vi "DisplayEndo.vi"(4 "Init?":bool, 5 "Hand Field Force":dbl[](array[numeric]), 6 "ClosePt":dbl[](array[numeric]), 7 "Tip Field Force":dbl[](array[numeric]), 8 "AnkleTraj":dbl[][](array[numeric]), 9 "Path Via Points":dbl[][](array[numeric])=[[0.0, 0.0, 0.0], [0.0, 0.0, 0.0], [0.0, 0.0, 0.0]], 10 "Joint Coord in GCS":dbl[][](array[numeric]), 11 "3D graph in":refnum<k7>) -> (3 "3D graph out":refnum<k7>)   [LabVIEW 2014]
uses:
  <vilib>/Platform/NI_3dgraph.lvlib
  <vilib>/ptbypt/NI_PtbyPt.lvlib
panel:
  in  "sample length":i32=100
  out "LastPlotNum":i32=1
  out "error out":errorcluster
  in  "error in (no error)":errorcluster
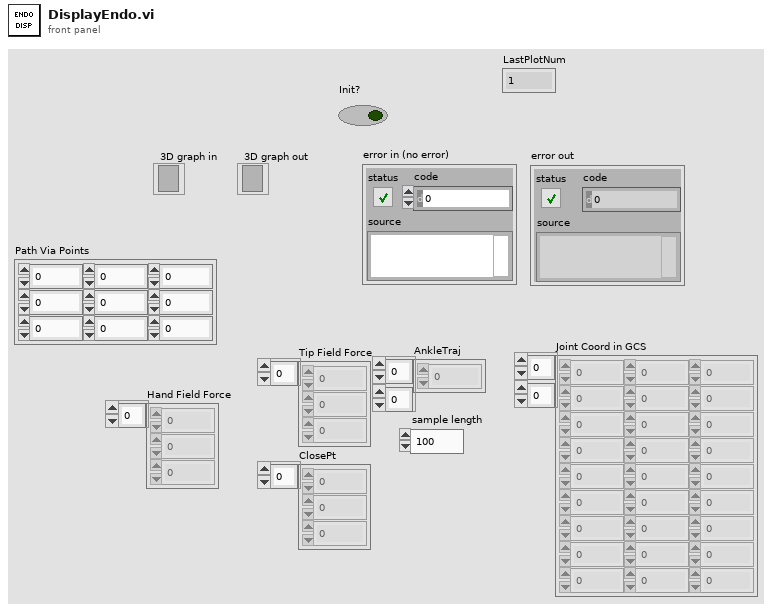
[diagram p1: front panel]
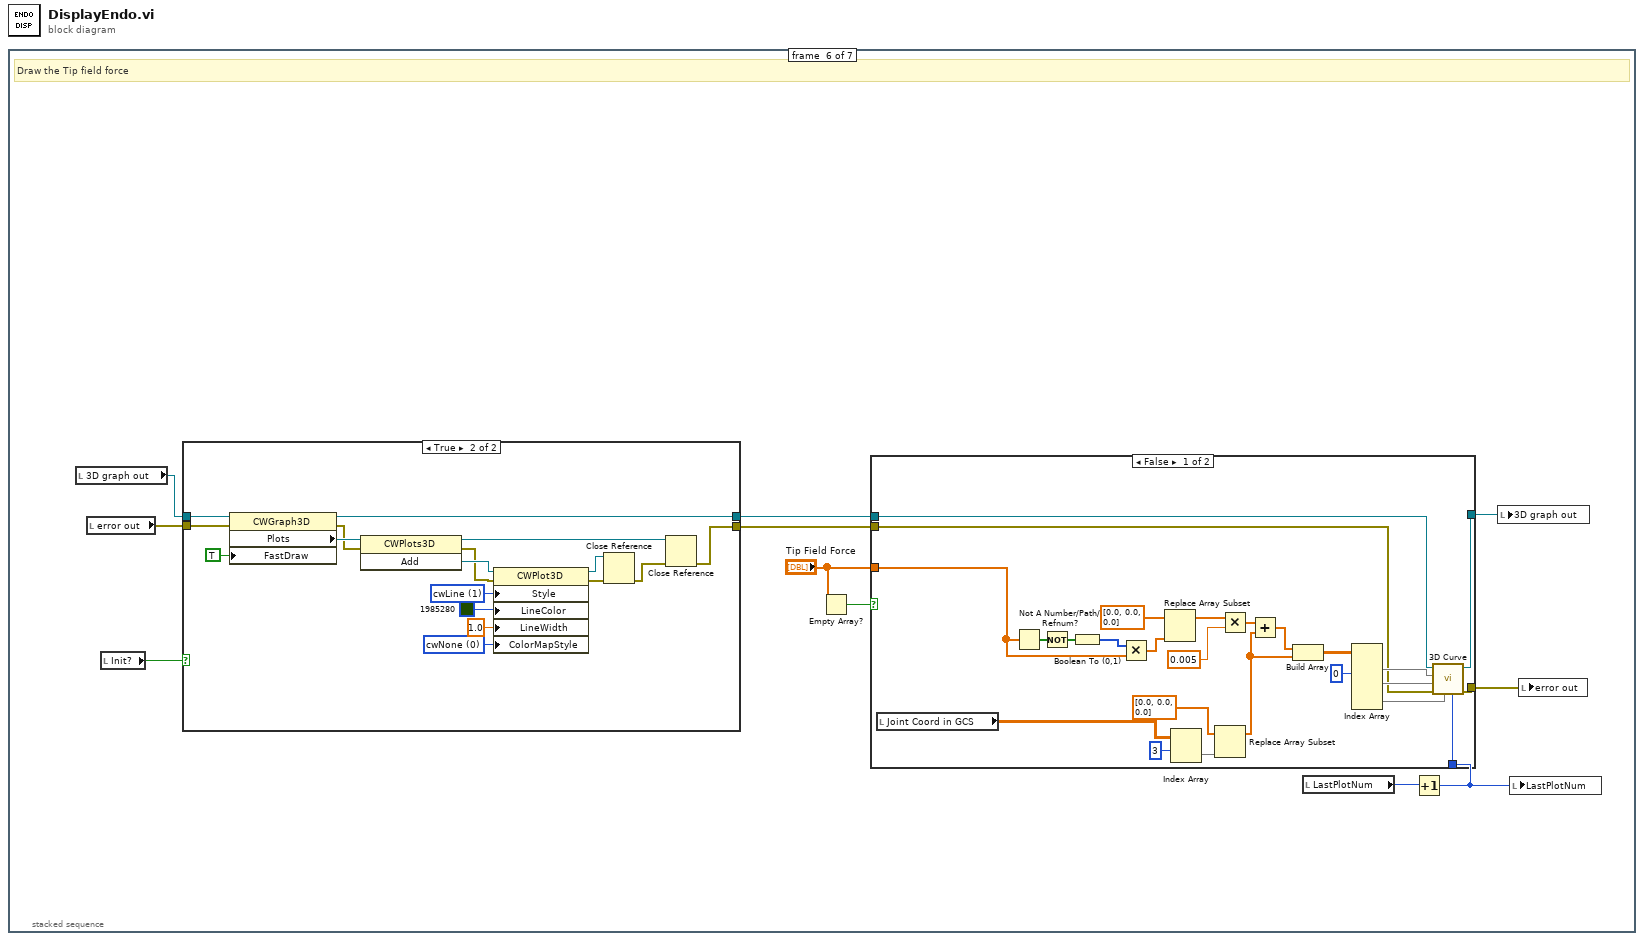
[diagram p0: block diagram]
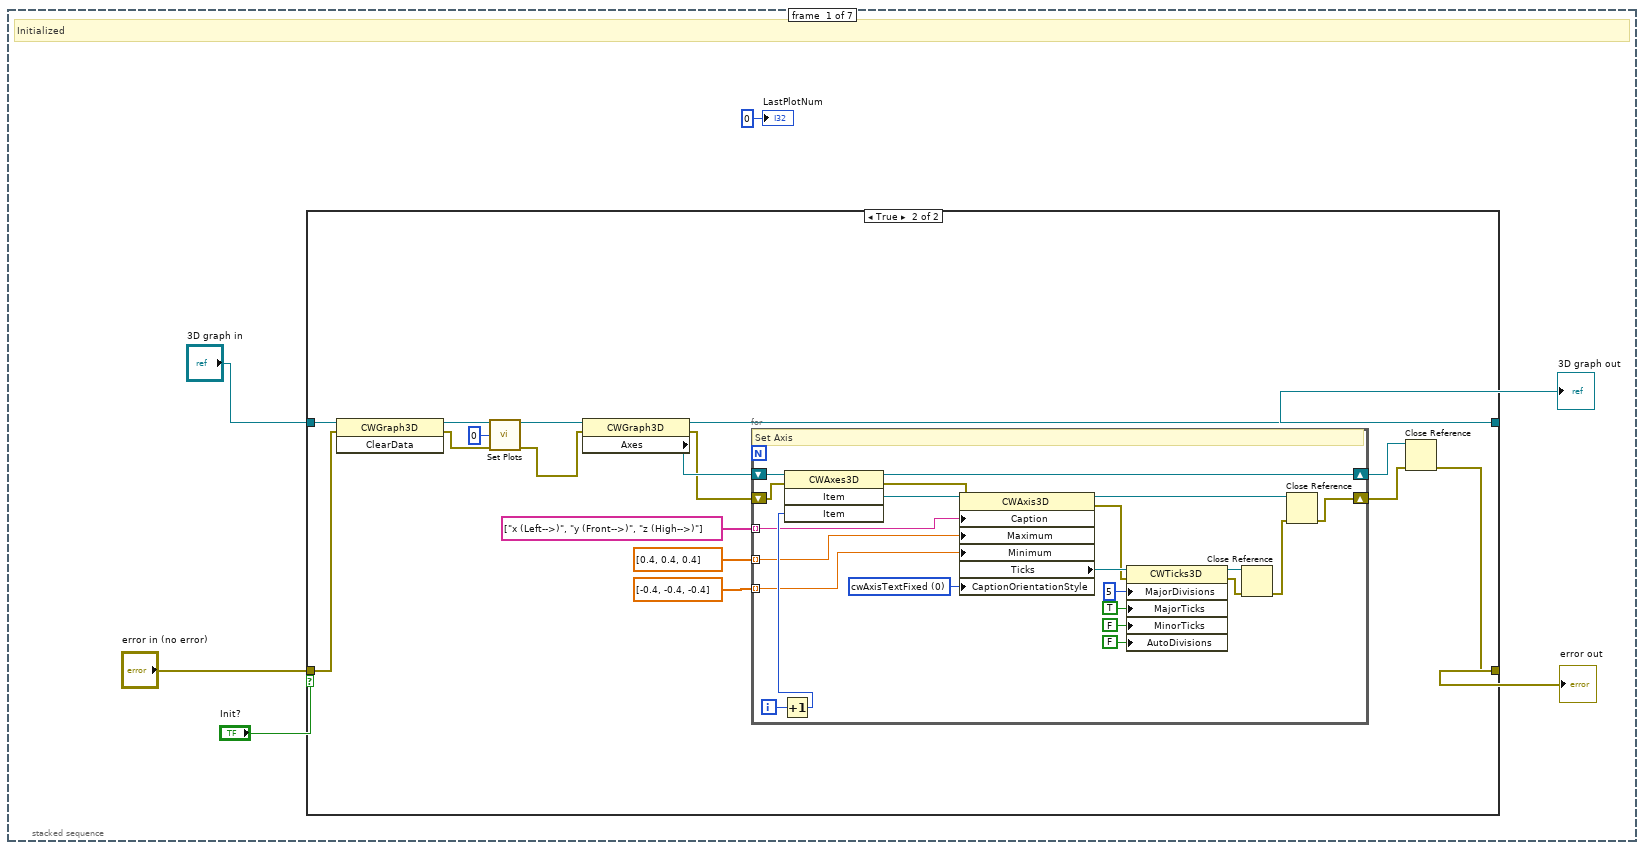
[diagram p2: hidden frame]
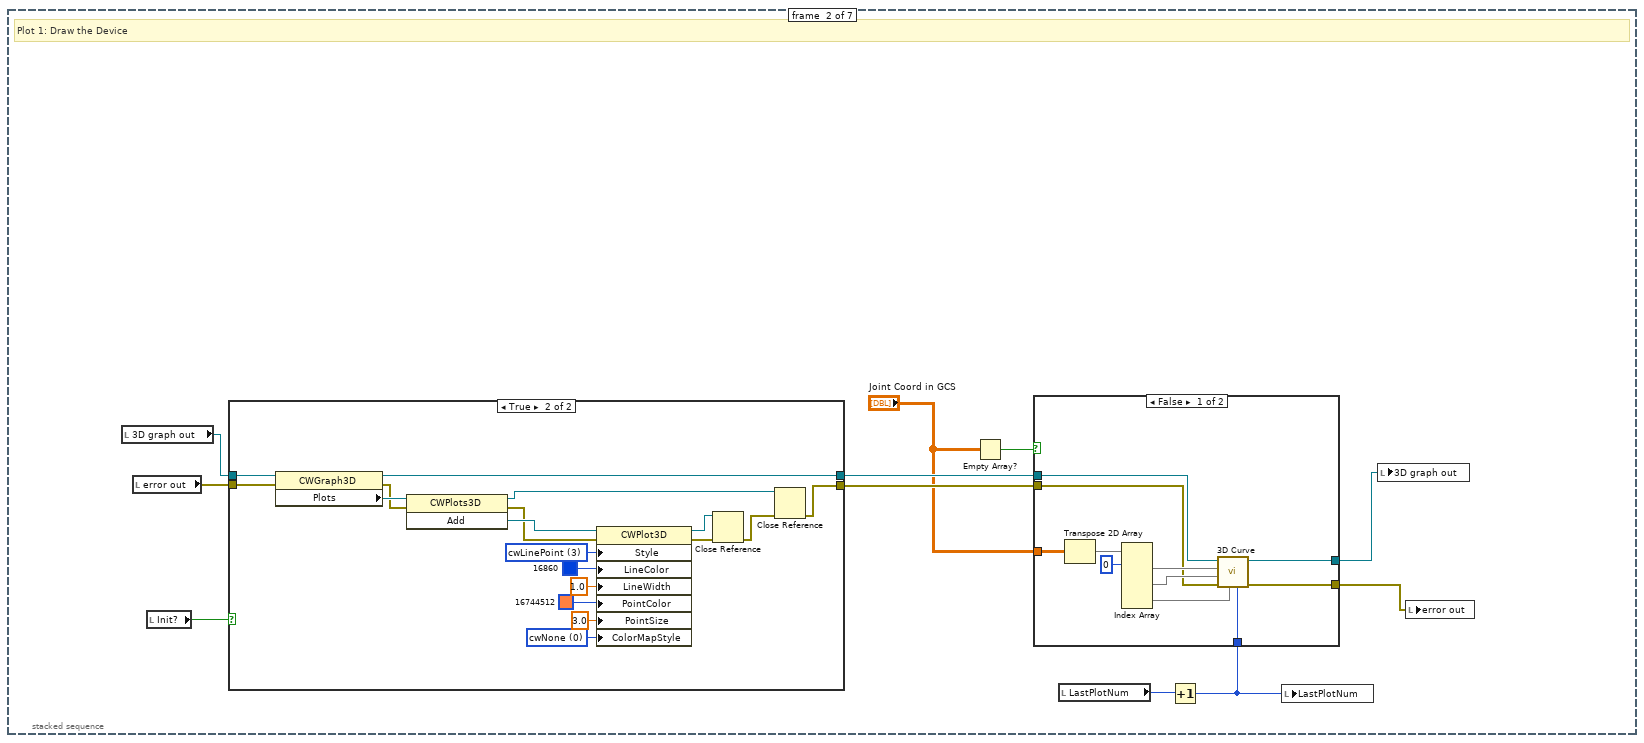
[diagram p4: hidden frame]
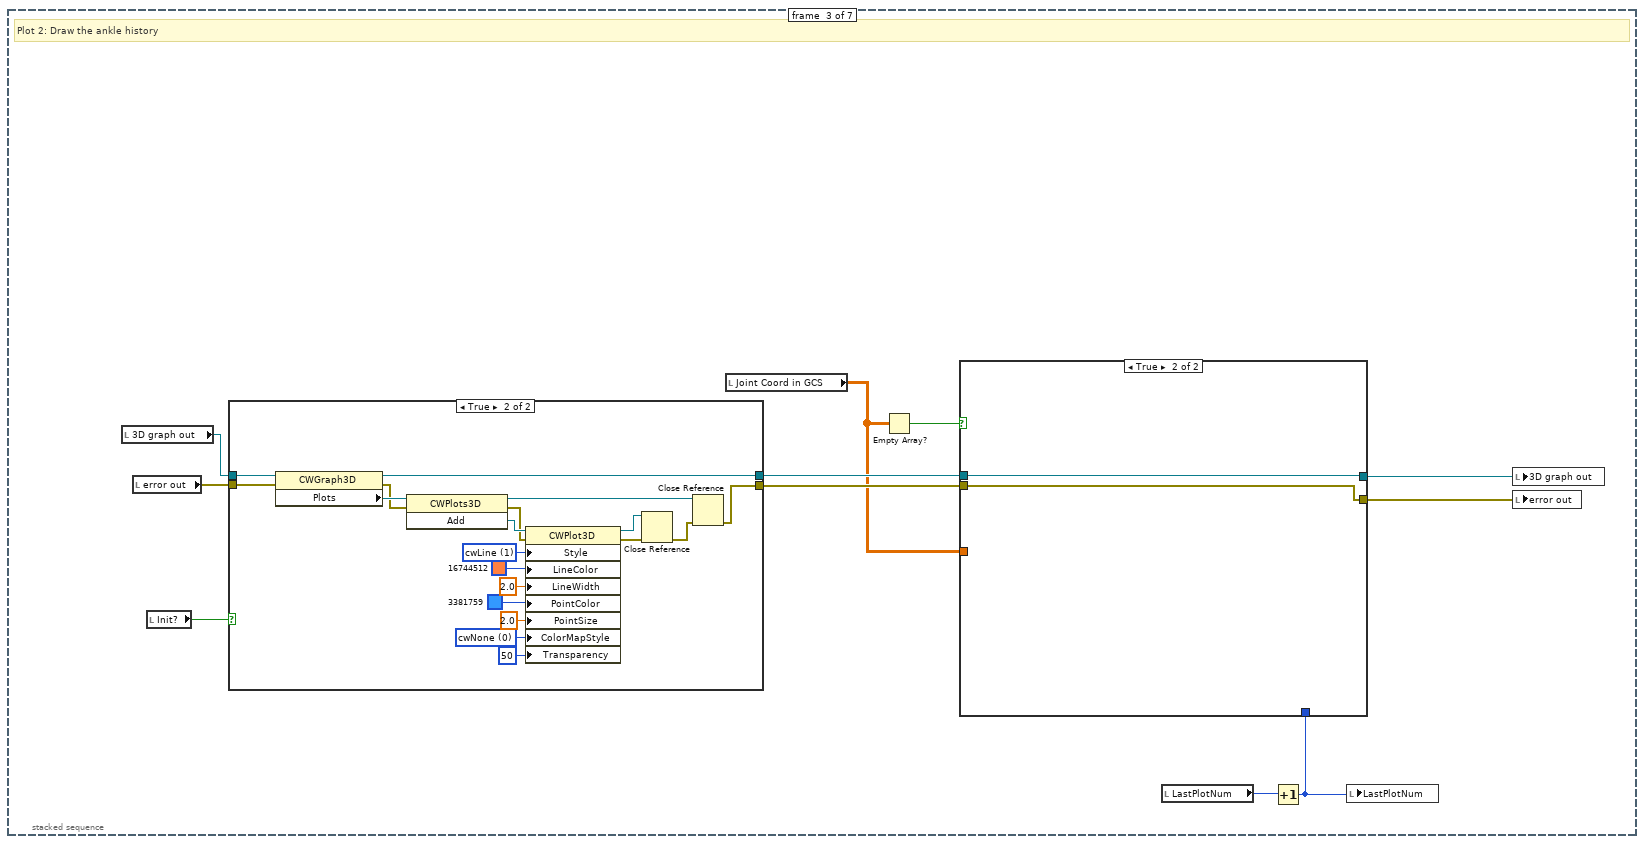
[diagram p7: hidden frame]
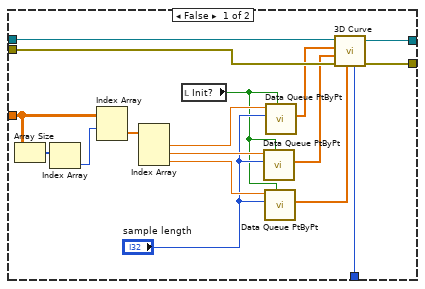
[diagram p8: hidden frame]
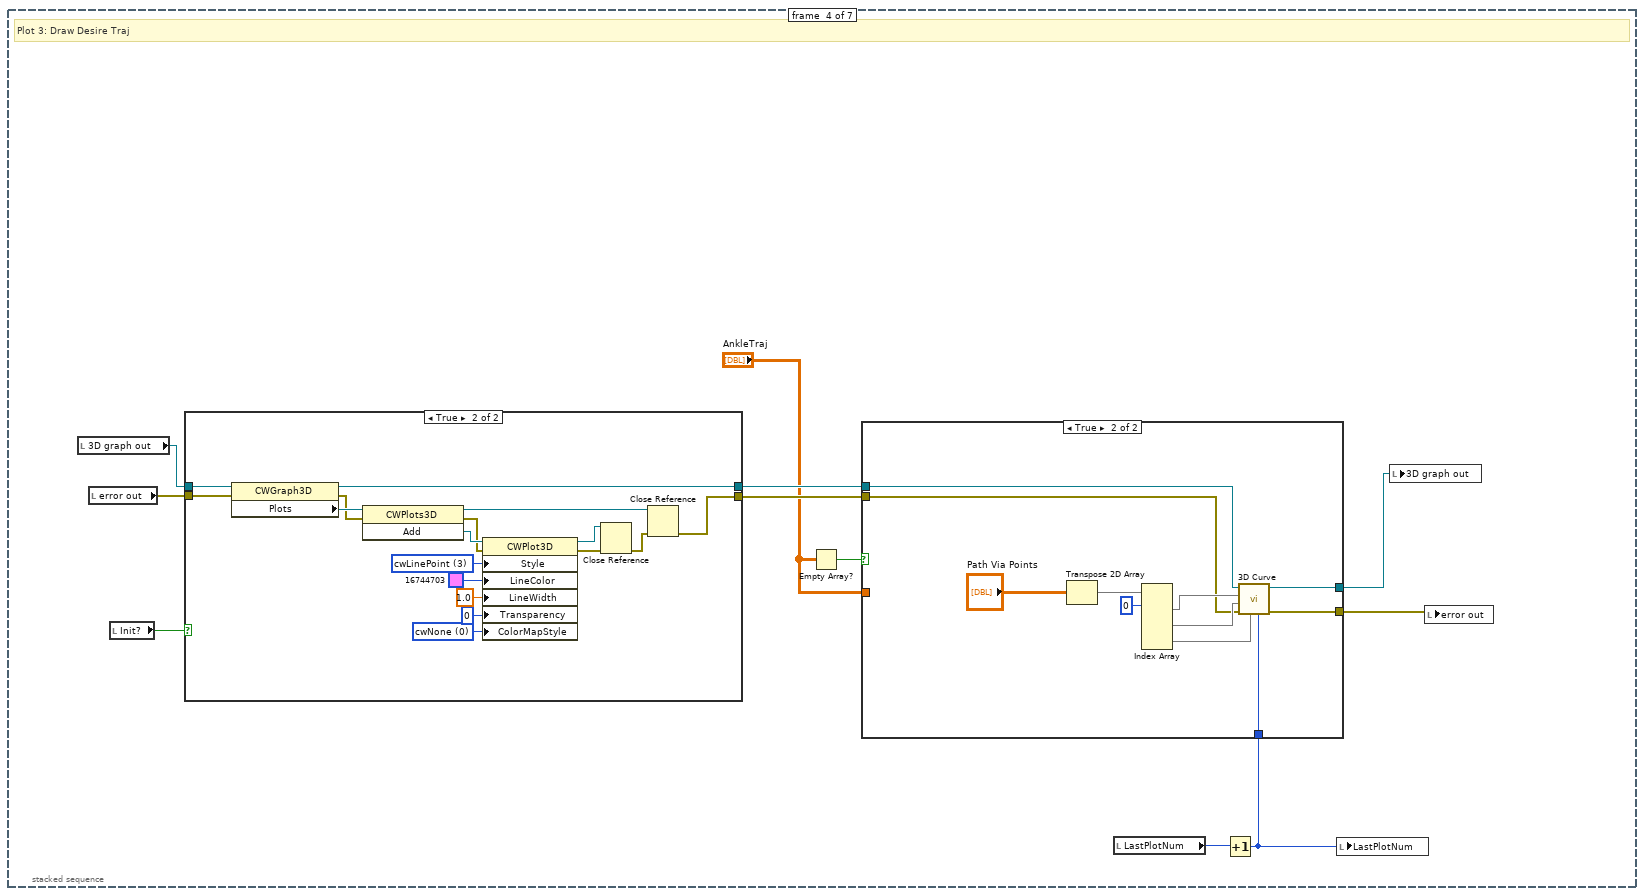
[diagram p10: hidden frame]
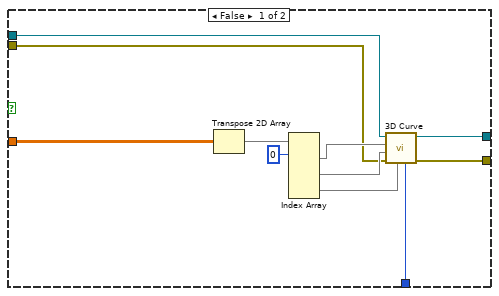
[diagram p11: hidden frame]
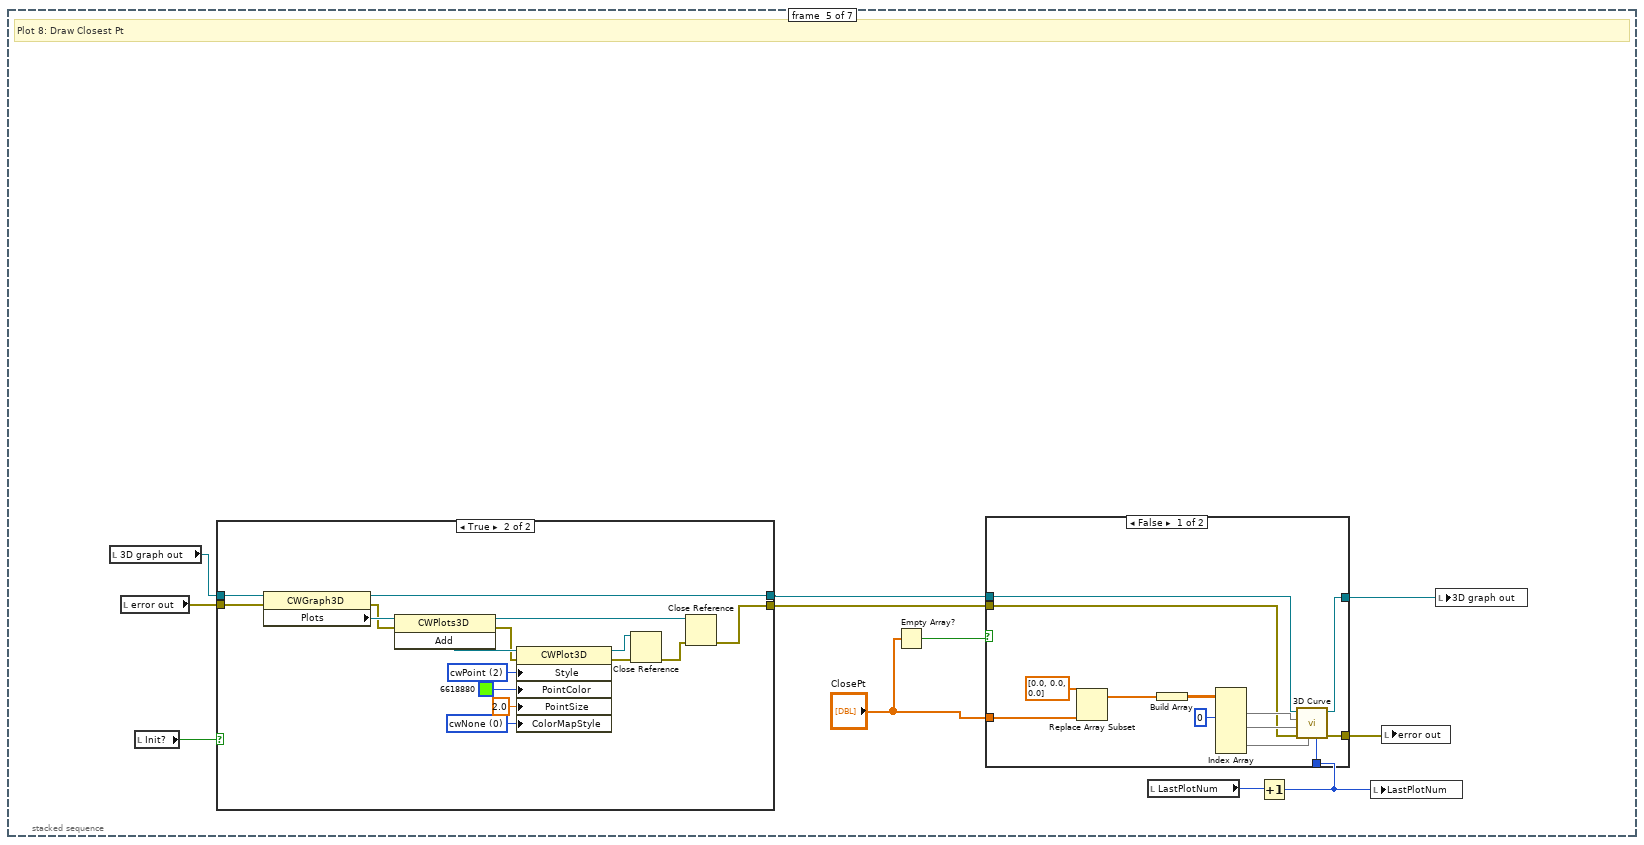
[diagram p13: hidden frame]
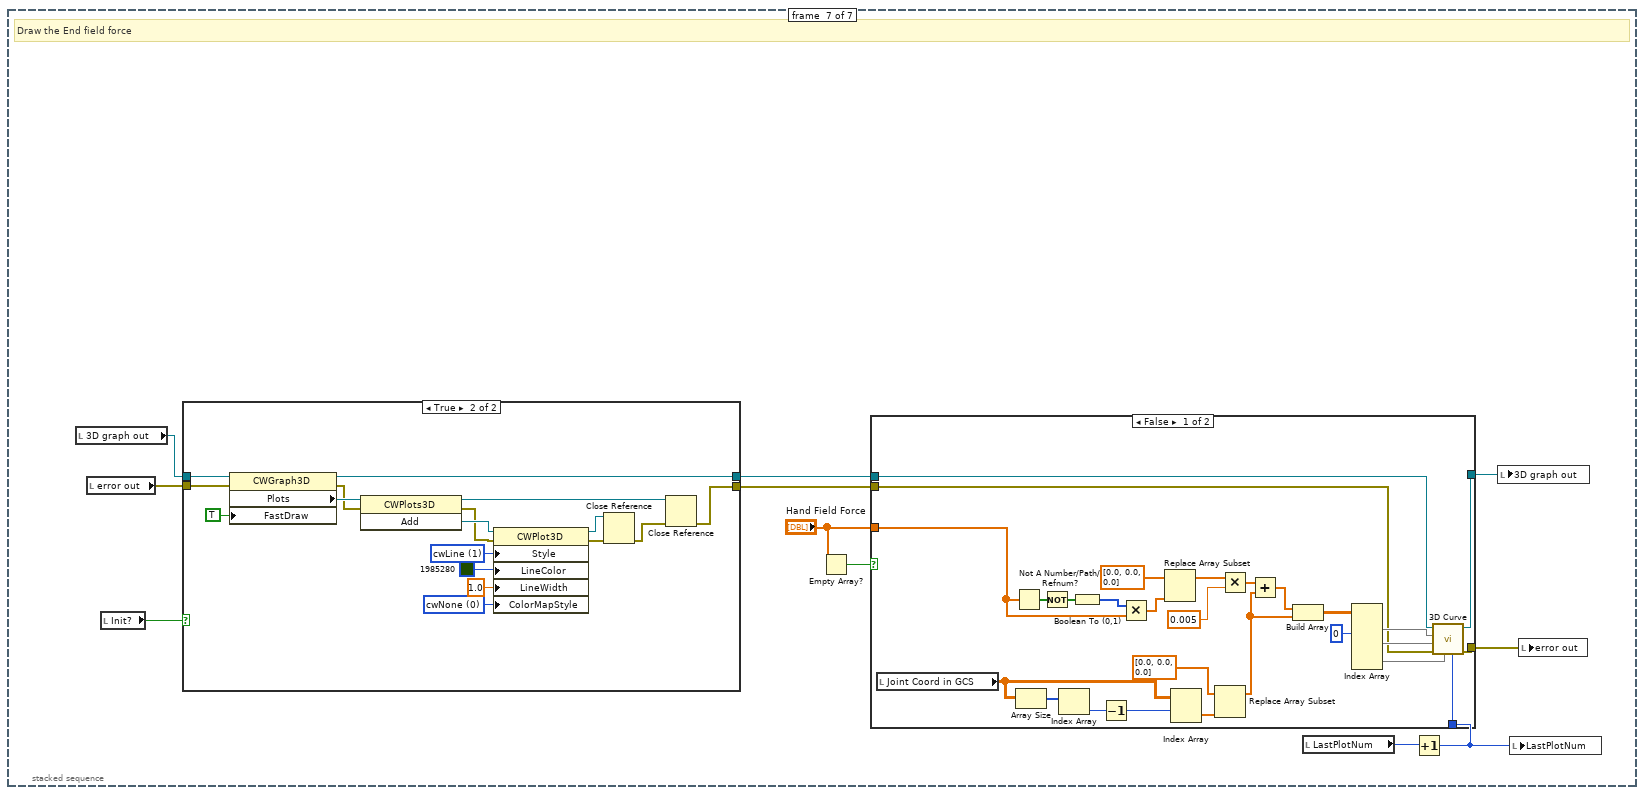
[diagram p18: hidden frame]
diagram:
  n1 = stacked-sequence {
    frame #0 {
      # "Initialized"
      n2 = case shown="True" "Init?" {
        tunnel: "3D graph in" -> [w8 w21]
        tunnel: [w8 w17] -> w5
        tunnel: [w7 w12] -> w3
        tunnel: "error in (no error)" -> [w7 w19]
        frame False {
        }
        frame True {
          n3 = invoke class="CWGraph3D" method="ClearData"(reference=w21, error in=w19) -> (reference out=w20:refnum<k7>, error out=w18:errorcluster)  [unwired: 1 in, 1 out]
          n4 = call <vilib>:"Set Plots.vi"("3D graph"=w20, "# of plots(1)"=0, "error in (no error)"=w18) -> ("3D graph out"=w22:refnum<k7>, "error out"=w13:errorcluster)  [unwired: 11 in]
          n5 = property class="CWGraph3D"(reference=w22, error in=w13) -> (reference out=w17:refnum<k7>, error out=w14:errorcluster, "Axes"=w23:refnum<k7>)
          n6 = for {
            shift-right: [w33] -> w15
            shift-left: w23 -> [w46]
            shift-right: [w34] -> w16
            shift-left: w14 -> [w31]
            tunnel: string[] ["x (Left-->)", "y (Front-->)", "z (High-->)"] -> [w27] mode=indexing
            tunnel: dbl[] [0.4, 0.4, 0.4] -> [w26] mode=indexing
            tunnel: dbl[] [-0.4, -0.4, -0.4] -> [w25] mode=indexing
            i -> [w29]
            w30 = 0 items=["cwAxisTextFixed", "cwAxisTextFaceCamera"] ("CaptionOrientationStyle")
            # "Set Axis"
            n7 = Increment(x=w29) -> (x+1=w28:i32)
            n8 = invoke class="CWAxes3D" method="Item"(reference=w46, error in=w31, "Item"=w28) -> (reference out=w33:refnum<k7>, error out=w32:errorcluster, "Item"=w45:refnum<k7>)  [unwired: 1 in, 1 out]
            n9 = property class="CWAxis3D"(reference=w45, error in=w32, "Caption"=w27, "Maximum"=w26, "Minimum"=w25, "CaptionOrientationStyle"=w30) -> (reference out=w35:refnum<k7>, error out=w38:errorcluster, "Ticks"=w44:refnum<k7>)
            n10 = property class="CWTicks3D"(reference=w44, error in=w38, "MajorDivisions"=5, "MajorTicks"=TRUE, "MinorTicks"=FALSE, "AutoDivisions"=FALSE) -> (reference out=w37:refnum<k7>, error out=w39:errorcluster)
            n11 = Close Reference(reference=w37, error in (no error)=w39) -> (error out=w36:errorcluster)
            n12 = Close Reference(reference=w35, error in (no error)=w36) -> (error out=w34:errorcluster)
          }
          n13 = Close Reference(reference=w15, error in (no error)=w16) -> (error out=w12:errorcluster)
        }
      }
      "3D graph out" <- w5
      "error out" <- w3
      "LastPlotNum" <- 0 ("LastPlotNum 2")
    }
    frame #1 {
      # "Plot 1: Draw the Device"
      n14 = local read "3D graph out"() -> (w55:refnum<k7>)
      n15 = local read "error out"() -> (w56:errorcluster)
      n16 = local read "Init?"() -> (w49:bool)
      n17 = case shown="True" w49 {
        tunnel: w56 -> [w71 w84]
        tunnel: w55 -> [w72 w79]
        tunnel: [w72 w78] -> w54
        tunnel: [w71 w73] -> w53
        frame False {
        }
        frame True {
          w77 = 0 items=["cwNone", "cwShaded", "cwColorSpectrum", "cwGrayScale", "cwCustom"] ("ColorMapStyle")
          w90 = 3 items=["cwLine"=1, "cwPoint"=2, "cwLinePoint"=3, "cwHiddenLine"=4, "cwSurface"=5, "cwSurfaceLine"=6, "cwSurfaceNormal"=7, "cwContourLine"=8, "cwSurfaceContour"=9] ("Style")
          n18 = property class="CWGraph3D"(reference=w79, error in=w84) -> (reference out=w78:refnum<k7>, error out=w87:errorcluster, "Plots"=w88:refnum<k7>)
          n19 = invoke class="CWPlots3D" method="Add"(reference=w88, error in=w87) -> (reference out=w75:refnum<k7>, error out=w76:errorcluster, "Add"=w89:refnum<k7>)  [unwired: 1 in]
          n20 = property class="CWPlot3D"(reference=w89, error in=w76, "Style"=w90, "LineColor"=u32 16860, "LineWidth"=1.0, "PointColor"=u32 16744512, "PointSize"=3.0 ("LineWidth"), "ColorMapStyle"=w77) -> (reference out=w85:refnum<k7>, error out=w86:errorcluster)
          n21 = Close Reference(reference=w85, error in (no error)=w86) -> (error out=w74:errorcluster)
          n22 = Close Reference(reference=w75, error in (no error)=w74) -> (error out=w73:errorcluster)
        }
      }
      n23 = Empty Array?(array="Joint Coord in GCS") -> (empty?=w47:bool)
      n24 = local read "LastPlotNum"() -> (w51:i32)
      n25 = Increment(x=w51) -> (x+1=w50:i32)
      n26 = case shown="False" w47 {
        tunnel: [w63 w70] -> w57
        tunnel: w54 -> [w62 w70]
        tunnel: w53 -> [w61 w69]
        tunnel: [w60 w69] -> w52
        tunnel: w50 -> [w59 _]
        tunnel: "Joint Coord in GCS" -> [w58 _]
        frame False {
          n27 = Transpose 2D Array(2D array=w58) -> (transposed array=w64:dbl[][])
          n28 = Index Array(array=w64, index (row) #1=0 ("index (row)")) -> (element #1=w66:dbl[], element #2=w67:dbl[], element #3=w68:dbl[])  [unwired: 5 in]
          n29 = call <vilib>:"3D Curve.vi"("plot number (1)"=w59, "z vector"=w68, "error in (no error)"=w61, "y vector"=w67, "x vector"=w66, "3D graph"=w62) -> ("error out"=w60:errorcluster, "3D graph out"=w63:refnum<k7>)  [unwired: 4 in]
        }
        frame True {
        }
      }
      n30 = local write "LastPlotNum"(w50) -> ()
      n31 = local write "3D graph out"(w57) -> ()
      n32 = local write "error out"(w52) -> ()
    }
    frame #2 {
      # "Plot 2: Draw the ankle history"
      n33 = local read "3D graph out"() -> (w99:refnum<k7>)
      n34 = local read "error out"() -> (w100:errorcluster)
      n35 = local read "Init?"() -> (w94:bool)
      n36 = case shown="True" w94 {
        tunnel: w100 -> [w121 w134]
        tunnel: w99 -> [w122 w129]
        tunnel: [w122 w128] -> w98
        tunnel: [w121 w123] -> w97
        frame False {
        }
        frame True {
          w127 = 0 items=["cwNone", "cwShaded", "cwColorSpectrum", "cwGrayScale", "cwCustom"] ("ColorMapStyle")
          w141 = 1 items=["cwLine"=1, "cwPoint"=2, "cwLinePoint"=3, "cwHiddenLine"=4, "cwSurface"=5, "cwSurfaceLine"=6, "cwSurfaceNormal"=7, "cwContourLine"=8, "cwSurfaceContour"=9] ("Style")
          n37 = property class="CWGraph3D"(reference=w129, error in=w134) -> (reference out=w128:refnum<k7>, error out=w138:errorcluster, "Plots"=w139:refnum<k7>)
          n38 = invoke class="CWPlots3D" method="Add"(reference=w139, error in=w138) -> (reference out=w137:refnum<k7>, error out=w125:errorcluster, "Add"=w140:refnum<k7>)  [unwired: 1 in]
          n39 = property class="CWPlot3D"(reference=w140, error in=w125, "Style"=w141, "LineColor"=u32 16744512, "LineWidth"=2.0, "PointColor"=u32 3381759, "PointSize"=2.0 ("LineWidth"), "ColorMapStyle"=w127, "Transparency"=50) -> (reference out=w135:refnum<k7>, error out=w136:errorcluster)
          n40 = Close Reference(reference=w135, error in (no error)=w136) -> (error out=w124:errorcluster)
          n41 = Close Reference(reference=w137, error in (no error)=w124) -> (error out=w123:errorcluster)
        }
      }
      n42 = local read "Joint Coord in GCS"() -> (w92:dbl[][])
      n43 = Empty Array?(array=w92) -> (empty?=w91:bool)
      n44 = local read "LastPlotNum"() -> (w93:i32)
      n45 = Increment(x=w93) -> (x+1=w95:i32)
      n46 = case shown="True" w91 {
        tunnel: [w118 w120] -> w101
        tunnel: w98 -> [w117 w120]
        tunnel: w97 -> [w116 w119]
        tunnel: [w115 w119] -> w96
        tunnel: w95 -> [w114 _]
        tunnel: w92 -> [w102 _]
        frame False {
          n47 = Array Size(array=w102) -> (size(s)=w113:i32[])
          n48 = Index Array(array=w113) -> (element=w112:i32)  [unwired: 1 in]
          n49 = Index Array(array=w102, index (row)=w112) -> (element=w111:dbl[])  [unwired: 1 in]
          n50 = Index Array(array=w111) -> (element #1=w108:dbl, element #2=w109:dbl, element #3=w110:dbl)  [unwired: 3 in]
          n51 = local read "Init?"() -> (w103:bool)
          n52 = call <vilib>:"Data Queue PtByPt.vi"("initialize"=w103, "sample length"="sample length", "input data point"=w109) -> ("Current Queue"=w105:dbl[])  [unwired: 4 in, 4 out]
          n53 = call <vilib>:"Data Queue PtByPt.vi"("initialize"=w103, "sample length"="sample length", "input data point"=w110) -> ("Current Queue"=w104:dbl[])  [unwired: 4 in, 4 out]
          n54 = call <vilib>:"Data Queue PtByPt.vi"("initialize"=w103, "sample length"="sample length", "input data point"=w108) -> ("Current Queue"=w106:dbl[])  [unwired: 4 in, 4 out]
          n55 = call <vilib>:"3D Curve.vi"("plot number (1)"=w114, "z vector"=w104, "error in (no error)"=w116, "y vector"=w105, "x vector"=w106, "3D graph"=w117) -> ("error out"=w115:errorcluster, "3D graph out"=w118:refnum<k7>)  [unwired: 4 in]
        }
        frame True {
        }
      }
      n56 = local write "LastPlotNum"(w95) -> ()
      n57 = local write "3D graph out"(w101) -> ()
      n58 = local write "error out"(w96) -> ()
    }
    frame #3 {
      # "Plot 3: Draw Desire Traj"
      n59 = local read "3D graph out"() -> (w150:refnum<k7>)
      n60 = local read "error out"() -> (w151:errorcluster)
      n61 = local read "Init?"() -> (w146:bool)
      n62 = case shown="True" w146 {
        tunnel: w151 -> [w175 w186]
        tunnel: w150 -> [w176 w183]
        tunnel: [w176 w182] -> w149
        tunnel: [w175 w177] -> w145
        frame False {
        }
        frame True {
          w180 = 0 items=["cwNone", "cwShaded", "cwColorSpectrum", "cwGrayScale", "cwCustom"] ("ColorMapStyle")
          w193 = 3 items=["cwLine"=1, "cwPoint"=2, "cwLinePoint"=3, "cwHiddenLine"=4, "cwSurface"=5, "cwSurfaceLine"=6, "cwSurfaceNormal"=7, "cwContourLine"=8, "cwSurfaceContour"=9] ("Style")
          n63 = property class="CWGraph3D"(reference=w183, error in=w186) -> (reference out=w182:refnum<k7>, error out=w190:errorcluster, "Plots"=w191:refnum<k7>)
          n64 = invoke class="CWPlots3D" method="Add"(reference=w191, error in=w190) -> (reference out=w189:refnum<k7>, error out=w179:errorcluster, "Add"=w192:refnum<k7>)  [unwired: 1 in]
          n65 = property class="CWPlot3D"(reference=w192, error in=w179, "Style"=w193, "LineColor"=u32 16744703, "LineWidth"=1.0, "Transparency"=0, "ColorMapStyle"=w180) -> (reference out=w187:refnum<k7>, error out=w188:errorcluster)
          n66 = Close Reference(reference=w187, error in (no error)=w188) -> (error out=w178:errorcluster)
          n67 = Close Reference(reference=w189, error in (no error)=w178) -> (error out=w177:errorcluster)
        }
      }
      n68 = Empty Array?(array="AnkleTraj") -> (empty?=w143:bool)
      n69 = local read "LastPlotNum"() -> (w148:i32)
      n70 = Increment(x=w148) -> (x+1=w147:i32)
      n71 = case shown="True" w143 {
        tunnel: "AnkleTraj" -> [w163 _]
        tunnel: [w157 w169] -> w152
        tunnel: w149 -> [w156 w168]
        tunnel: w147 -> [w155 w167]
        tunnel: w145 -> [w154 w166]
        tunnel: [w153 w165] -> w144
        frame False {
          n72 = Transpose 2D Array(2D array=w163) -> (transposed array=w158:dbl[][])
          n73 = Index Array(array=w158, index (row) #1=0 ("index (row)")) -> (element #1=w160:dbl[], element #2=w161:dbl[], element #3=w162:dbl[])  [unwired: 5 in]
          n74 = call <vilib>:"3D Curve.vi"("plot number (1)"=w155, "z vector"=w162, "error in (no error)"=w154, "y vector"=w161, "x vector"=w160, "3D graph"=w156) -> ("error out"=w153:errorcluster, "3D graph out"=w157:refnum<k7>)  [unwired: 4 in]
        }
        frame True {
          n75 = Transpose 2D Array(2D array="Path Via Points") -> (transposed array=w170:dbl[][])
          n76 = Index Array(array=w170, index (row) #1=0 ("index (row)")) -> (element #1=w172:dbl[], element #2=w173:dbl[], element #3=w174:dbl[])  [unwired: 5 in]
          n77 = call <vilib>:"3D Curve.vi"("plot number (1)"=w167, "z vector"=w174, "error in (no error)"=w166, "y vector"=w173, "x vector"=w172, "3D graph"=w168) -> ("error out"=w165:errorcluster, "3D graph out"=w169:refnum<k7>)  [unwired: 4 in]
        }
      }
      n78 = local write "LastPlotNum"(w147) -> ()
      n79 = local write "3D graph out"(w152) -> ()
      n80 = local write "error out"(w144) -> ()
    }
    frame #4 {
      # "Plot 8: Draw Closest Pt"
      n81 = local read "3D graph out"() -> (w202:refnum<k7>)
      n82 = local read "error out"() -> (w203:errorcluster)
      n83 = local read "Init?"() -> (w201:bool)
      n84 = case shown="True" w201 {
        tunnel: w203 -> [w220 w230]
        tunnel: w202 -> [w221 w227]
        tunnel: [w221 w226] -> w200
        tunnel: [w220 w222] -> w197
        frame False {
        }
        frame True {
          w225 = 0 items=["cwNone", "cwShaded", "cwColorSpectrum", "cwGrayScale", "cwCustom"] ("ColorMapStyle")
          w237 = 2 items=["cwLine"=1, "cwPoint"=2, "cwLinePoint"=3, "cwHiddenLine"=4, "cwSurface"=5, "cwSurfaceLine"=6, "cwSurfaceNormal"=7, "cwContourLine"=8, "cwSurfaceContour"=9] ("Style")
          n85 = property class="CWGraph3D"(reference=w227, error in=w230) -> (reference out=w226:refnum<k7>, error out=w234:errorcluster, "Plots"=w235:refnum<k7>)
          n86 = invoke class="CWPlots3D" method="Add"(reference=w235, error in=w234) -> (reference out=w233:refnum<k7>, error out=w224:errorcluster, "Add"=w236:refnum<k7>)  [unwired: 1 in]
          n87 = property class="CWPlot3D"(reference=w236, error in=w224, "Style"=w237, "PointColor"=u32 6618880, "PointSize"=2.0 ("LineWidth"), "ColorMapStyle"=w225) -> (reference out=w231:refnum<k7>, error out=w232:errorcluster)
          n88 = Close Reference(reference=w231, error in (no error)=w232) -> (error out=w223:errorcluster)
          n89 = Close Reference(reference=w233, error in (no error)=w223) -> (error out=w222:errorcluster)
        }
      }
      n90 = Empty Array?(array="ClosePt") -> (empty?=w194:bool)
      n91 = local read "LastPlotNum"() -> (w199:i32)
      n92 = Increment(x=w199) -> (x+1=w198:i32)
      n93 = case shown="False" w194 {
        tunnel: "ClosePt" -> [w216 _]
        tunnel: [w209 w219] -> w204
        tunnel: w200 -> [w208 w219]
        tunnel: w198 -> [w207 _]
        tunnel: w197 -> [w206 w218]
        tunnel: [w205 w218] -> w196
        frame False {
          n94 = Replace Array Subset(array=dbl[] [0.0, 0.0, 0.0], new element=w216) -> (w215:dbl[])  [unwired: 1 in]
          n95 = Build Array(w215) -> (w214:dbl[][])
          n96 = Index Array(array=w214, index (col) #1=0 ("disabled index (col)")) -> (element #1=w212:dbl[], element #2=w211:dbl[], element #3=w210:dbl[])  [unwired: 5 in]
          n97 = call <vilib>:"3D Curve.vi"("plot number (1)"=w207, "z vector"=w210, "error in (no error)"=w206, "y vector"=w211, "x vector"=w212, "3D graph"=w208) -> ("error out"=w205:errorcluster, "3D graph out"=w209:refnum<k7>)  [unwired: 4 in]
        }
        frame True {
        }
      }
      n98 = local write "LastPlotNum"(w198) -> ()
      n99 = local write "error out"(w196) -> ()
      n100 = local write "3D graph out"(w204) -> ()
    }
    frame #5 {
      # "Draw the Tip field force"
      n101 = local read "3D graph out"() -> (w246:refnum<k7>)
      n102 = local read "error out"() -> (w247:errorcluster)
      n103 = local read "Init?"() -> (w245:bool)
      n104 = case shown="True" w245 {
        tunnel: w247 -> [w276 w287]
        tunnel: w246 -> [w277 w284]
        tunnel: [w277 w283] -> w244
        tunnel: [w276 w278] -> w241
        frame False {
        }
        frame True {
          w282 = 0 items=["cwNone", "cwShaded", "cwColorSpectrum", "cwGrayScale", "cwCustom"] ("ColorMapStyle")
          w294 = 1 items=["cwLine"=1, "cwPoint"=2, "cwLinePoint"=3, "cwHiddenLine"=4, "cwSurface"=5, "cwSurfaceLine"=6, "cwSurfaceNormal"=7, "cwContourLine"=8, "cwSurfaceContour"=9] ("Style")
          n105 = property class="CWGraph3D"(reference=w284, error in=w287, "FastDraw"=TRUE) -> (reference out=w283:refnum<k7>, error out=w291:errorcluster, "Plots"=w292:refnum<k7>)
          n106 = invoke class="CWPlots3D" method="Add"(reference=w292, error in=w291) -> (reference out=w290:refnum<k7>, error out=w280:errorcluster, "Add"=w293:refnum<k7>)  [unwired: 1 in]
          n107 = property class="CWPlot3D"(reference=w293, error in=w280, "Style"=w294, "LineColor"=u32 1985280, "LineWidth"=1.0, "ColorMapStyle"=w282) -> (reference out=w288:refnum<k7>, error out=w289:errorcluster)
          n108 = Close Reference(reference=w288, error in (no error)=w289) -> (error out=w279:errorcluster)
          n109 = Close Reference(reference=w290, error in (no error)=w279) -> (error out=w278:errorcluster)
        }
      }
      n110 = Empty Array?(array="Tip Field Force") -> (empty?=w238:bool)
      n111 = local read "LastPlotNum"() -> (w243:i32)
      n112 = Increment(x=w243) -> (x+1=w242:i32)
      n113 = case shown="False" w238 {
        tunnel: [w255 w275] -> w248
        tunnel: w244 -> [w254 w275]
        tunnel: w242 -> [w253 _]
        tunnel: w241 -> [w252 w274]
        tunnel: [w251 w274] -> w240
        tunnel: "Tip Field Force" -> [w250 _]
        frame False {
          n114 = local read "Joint Coord in GCS"() -> (w273:dbl[][])
          n115 = Not A Number/Path/Refnum?(number/path/refnum=w250) -> (NaN/Path/Refnum?=w259:bool[])
          n116 = Not(x=w259) -> (.not. x?=w258:bool[])
          n117 = Boolean To (0,1)(Boolean=w258) -> (0, 1=w257:i16[])
          n118 = Multiply(x=w257, y=w250) -> (x*y=w256:dbl[])
          n119 = Replace Array Subset(array=dbl[] [0.0, 0.0, 0.0], new element=w256) -> (w269:dbl[])  [unwired: 1 in]
          n120 = Index Array(array=w273, index (row)=3) -> (element=w271:dbl[])  [unwired: 1 in]
          n121 = Replace Array Subset(array=dbl[] [0.0, 0.0, 0.0], new element=w271) -> (w272:dbl[])  [unwired: 1 in]
          n122 = Multiply(x=w269, y=0.005) -> (x*y=w264:dbl[])
          n123 = Add(x=w264, y=w272) -> (x+y=w261:dbl[])
          n124 = Build Array(w261, w272) -> (w262:dbl[][])
          n125 = Index Array(array=w262, index (col) #1=0 ("disabled index (col)")) -> (element #1=w265:dbl[], element #2=w266:dbl[], element #3=w267:dbl[])  [unwired: 5 in]
          n126 = call <vilib>:"3D Curve.vi"("plot number (1)"=w253, "z vector"=w267, "error in (no error)"=w252, "y vector"=w266, "x vector"=w265, "3D graph"=w254) -> ("error out"=w251:errorcluster, "3D graph out"=w255:refnum<k7>)  [unwired: 4 in]
        }
        frame True {
        }
      }
      n127 = local write "3D graph out"(w248) -> ()
      n128 = local write "LastPlotNum"(w242) -> ()
      n129 = local write "error out"(w240) -> ()
    }
    frame #6 {
      # "Draw the End field force"
      n130 = local read "3D graph out"() -> (w303:refnum<k7>)
      n131 = local read "error out"() -> (w304:errorcluster)
      n132 = local read "Init?"() -> (w302:bool)
      n133 = case shown="True" w302 {
        tunnel: w304 -> [w335 w346]
        tunnel: w303 -> [w336 w343]
        tunnel: [w336 w342] -> w301
        tunnel: [w335 w337] -> w298
        frame False {
        }
        frame True {
          w341 = 0 items=["cwNone", "cwShaded", "cwColorSpectrum", "cwGrayScale", "cwCustom"] ("ColorMapStyle")
          w353 = 1 items=["cwLine"=1, "cwPoint"=2, "cwLinePoint"=3, "cwHiddenLine"=4, "cwSurface"=5, "cwSurfaceLine"=6, "cwSurfaceNormal"=7, "cwContourLine"=8, "cwSurfaceContour"=9] ("Style")
          n134 = property class="CWGraph3D"(reference=w343, error in=w346, "FastDraw"=TRUE) -> (reference out=w342:refnum<k7>, error out=w350:errorcluster, "Plots"=w351:refnum<k7>)
          n135 = invoke class="CWPlots3D" method="Add"(reference=w351, error in=w350) -> (reference out=w349:refnum<k7>, error out=w339:errorcluster, "Add"=w352:refnum<k7>)  [unwired: 1 in]
          n136 = property class="CWPlot3D"(reference=w352, error in=w339, "Style"=w353, "LineColor"=u32 1985280, "LineWidth"=1.0, "ColorMapStyle"=w341) -> (reference out=w347:refnum<k7>, error out=w348:errorcluster)
          n137 = Close Reference(reference=w347, error in (no error)=w348) -> (error out=w338:errorcluster)
          n138 = Close Reference(reference=w349, error in (no error)=w338) -> (error out=w337:errorcluster)
        }
      }
      n139 = Empty Array?(array="Hand Field Force") -> (empty?=w295:bool)
      n140 = local read "LastPlotNum"() -> (w300:i32)
      n141 = Increment(x=w300) -> (x+1=w299:i32)
      n142 = case shown="False" w295 {
        tunnel: [w312 w334] -> w305
        tunnel: w301 -> [w311 w334]
        tunnel: w299 -> [w310 _]
        tunnel: w298 -> [w309 w333]
        tunnel: [w308 w333] -> w297
        tunnel: "Hand Field Force" -> [w307 _]
        frame False {
          n143 = local read "Joint Coord in GCS"() -> (w332:dbl[][])
          n144 = Not A Number/Path/Refnum?(number/path/refnum=w307) -> (NaN/Path/Refnum?=w316:bool[])
          n145 = Array Size(array=w332) -> (size(s)=w322:i32[])
          n146 = Not(x=w316) -> (.not. x?=w315:bool[])
          n147 = Index Array(array=w322) -> (element=w323:i32)  [unwired: 1 in]
          n148 = Boolean To (0,1)(Boolean=w315) -> (0, 1=w314:i16[])
          n149 = Decrement(x=w323) -> (x-1=w306:i32)
          n150 = Multiply(x=w314, y=w307) -> (x*y=w313:dbl[])
          n151 = Replace Array Subset(array=dbl[] [0.0, 0.0, 0.0], new element=w313) -> (w328:dbl[])  [unwired: 1 in]
          n152 = Index Array(array=w332, index (row)=w306) -> (element=w330:dbl[])  [unwired: 1 in]
          n153 = Replace Array Subset(array=dbl[] [0.0, 0.0, 0.0], new element=w330) -> (w331:dbl[])  [unwired: 1 in]
          n154 = Multiply(x=w328, y=0.005) -> (x*y=w321:dbl[])
          n155 = Add(x=w321, y=w331) -> (x+y=w318:dbl[])
          n156 = Build Array(w318, w331) -> (w319:dbl[][])
          n157 = Index Array(array=w319, index (col) #1=0 ("disabled index (col)")) -> (element #1=w324:dbl[], element #2=w325:dbl[], element #3=w326:dbl[])  [unwired: 5 in]
          n158 = call <vilib>:"3D Curve.vi"("plot number (1)"=w310, "z vector"=w326, "error in (no error)"=w309, "y vector"=w325, "x vector"=w324, "3D graph"=w311) -> ("error out"=w308:errorcluster, "3D graph out"=w312:refnum<k7>)  [unwired: 4 in]
        }
        frame True {
        }
      }
      n159 = local write "3D graph out"(w305) -> ()
      n160 = local write "LastPlotNum"(w299) -> ()
      n161 = local write "error out"(w297) -> ()
    }
  }
